vi "ExtractImagePlane.vi"(1 "Router":u32, 2 "Plane":u32, 3 "Trace":u32[][][][](array[numeric])) -> (0 "Intensity":u32[][](array[numeric]))   [LabVIEW 2009]
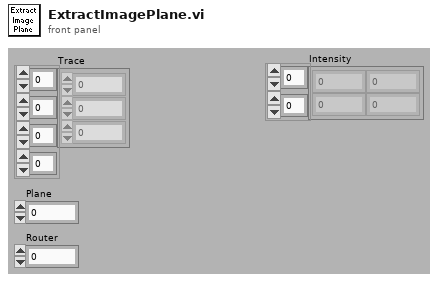
[diagram p1: front panel]
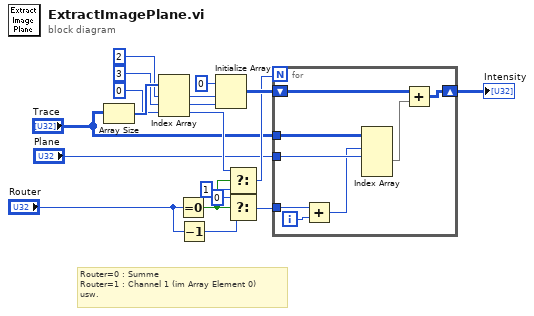
[diagram p0: block diagram]
diagram:
  # "Router=0 : Summe\nRouter=1 : Channel 1 (im Array Element 0)\nusw."
  n1 = Array Size(array="Trace") -> (size(s)=w17:i32[])
  n2 = Index Array(array=w17, index #1=2 ("index"), index #2=3 ("index"), index #3=0 ("index")) -> (element #1=w14:i32, element #2=w13:i32, element #3=w10:i32)
  n3 = Equal To 0?(x="Router") -> (x = 0?=w9:bool)
  n4 = Decrement(x="Router") -> (x-1=w2:u32)
  n5 = Initialize Array(u32 0, w14, w13) -> (w18:u32[][])
  n6 = Select(t=w10, s=w9, f=1) -> (s? t:f=w12:i32)
  n7 = Select(t=u32 0, s=w9, f=w2) -> (s? t:f=w7:u32)
  n8 = for {
    N: w12 -> [_]
    tunnel: "Trace" -> [w27]
    tunnel: "Plane" -> [w23]
    shift-right: [w24] -> w3
    shift-left: w18 -> [w25]
    tunnel: w7 -> [w22]
    i -> [w21]
    n9 = Add(x=w22, y=w21) -> (x+y=w20:u32)
    n10 = Index Array(array=w27, index (dim 0)=w20, index (dim 1)=w23) -> (element=w26:u32[][])  [unwired: 2 in]
    n11 = Add(x=w25, y=w26) -> (x+y=w24:u32[][])
  }
  "Intensity" <- w3
